vi "Output Protection Status.vi"(8 "error in (no error)":errorcluster, 11 "VISA resource name":refnum<visa-resource-name>) -> (0 "error out":errorcluster, 1 "OCP Tripped?":bool, 2 "OVP Tripped?":bool, 3 "VISA resource name out":refnum<visa-resource-name>)   [LabVIEW 2020, in "Agilent E363X Series.lvlib"]
doc: "Returns Over Voltage Protection (OVP) and Over Current Protection (OCP) status for a desired channel.\n\n<B>Note:</B> OVP/OCP not supported on E3631"
uses:
  Agilent E363X Series.lvlib
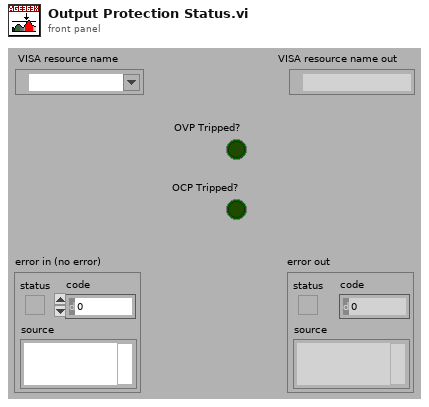
[diagram p1: front panel]
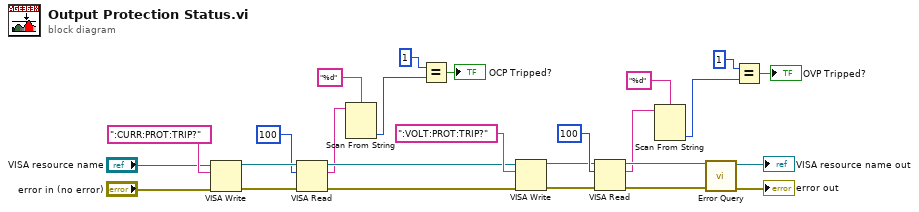
[diagram p0: block diagram]
diagram:
  n1 = VISA Write(VISA resource name="VISA resource name", write buffer=":CURR:PROT:TRIP?", error in (no error)="error in (no error)") -> (VISA resource name out=w22:refnum<visa-resource-name>, error out=w23:errorcluster)  [unwired: 1 out]
  n2 = VISA Read(VISA resource name=w22, byte count=u32 100, error in (no error)=w23) -> (VISA resource name out=w14:refnum<visa-resource-name>, read buffer=w10:string, error out=w13:errorcluster)  [unwired: 1 out]
  n3 = Scan From String(format string="%d", input string=w10) -> (output 1=w4:i32)  [unwired: 3 in, 3 out]
  n4 = Equal?(x=1, y=w4) -> (x = y?=→"OCP Tripped?":bool)
  n5 = VISA Write(VISA resource name=w14, write buffer=":VOLT:PROT:TRIP?", error in (no error)=w13) -> (VISA resource name out=w18:refnum<visa-resource-name>, error out=w17:errorcluster)  [unwired: 1 out]
  n6 = VISA Read(VISA resource name=w18, byte count=u32 100, error in (no error)=w17) -> (VISA resource name out=w12:refnum<visa-resource-name>, read buffer=w6:string, error out=w11:errorcluster)  [unwired: 1 out]
  n7 = Scan From String(format string="%d", input string=w6) -> (output 1=w3:i32)  [unwired: 3 in, 3 out]
  n8 = call "Error Query.vi"("error in (no error)"=w11, "VISA resource name"=w12) -> ("error out"=→"error out":errorcluster, "VISA resource name out"=→"VISA resource name out":refnum<visa-resource-name>)  [unwired: 6 in, 2 out]
  n9 = Equal?(x=1, y=w3) -> (x = y?=→"OVP Tripped?":bool)
